vi "AM Modulation Demo (Baseband-Sine) - multi.vi"() -> ()   [LabVIEW 2013]
uses:
  <vilib>/express/express analysis/Spectral/Block/exnSpectralBlock spectral measurements power poly.vi
  <vilib>/express/express analysis/Spectral/Block/exnSpectralBlock spectral measurements power DDT.vi
  <vilib>/express/express analysis/Spectral/XNode/ExpressSpectralMeasurementsBlockNode.xnode
panel:
  in  "Noise Deviation":dbl=0.1 caption="Amplitude"
  out "After Filter 2":dynamicdata(graph)
  out "Baseband 2":dynamicdata(graph)
  out "Comparision 2":dynamicdata(graph)
  in  "DC Offset 2":dbl=1.0
  in  "Carrier Amp. 2":dbl=1.0 caption="Amplitude"
  in  "Carrier Freq. 2":dbl=100000.0 caption="Frequency"
  in  "Modulation Index 2":dbl(slide)=1.0 scale=0.0..5.0
  in  "Mod Freq. 2":dbl=1000.0 caption="Frequency"
  out "After Filter 1":dynamicdata(graph)
  in  "Mod Freq.":dbl=2000.0 caption="Frequency"
  in  "LPF Cut-Off":dbl=10000.0 caption="Lower Cut-Off"
  out "Comparision 1":dynamicdata(graph)
  out "Baseband 1":dynamicdata(graph)
  out "AM Power Spectrum":dynamicdata(graph)
  out "AM Wave":dynamicdata(graph)
  in  "DC Offset":dbl=1.0
  in  "Carrier Amp.":dbl=1.0 caption="Amplitude"
  in  "stop":bool
  in  "Modulation Index":dbl(slide)=1.0 scale=0.0..5.0
  in  "Carrier Freq.":dbl=50000.0 caption="Frequency"
  # "Amplitude Modulation"
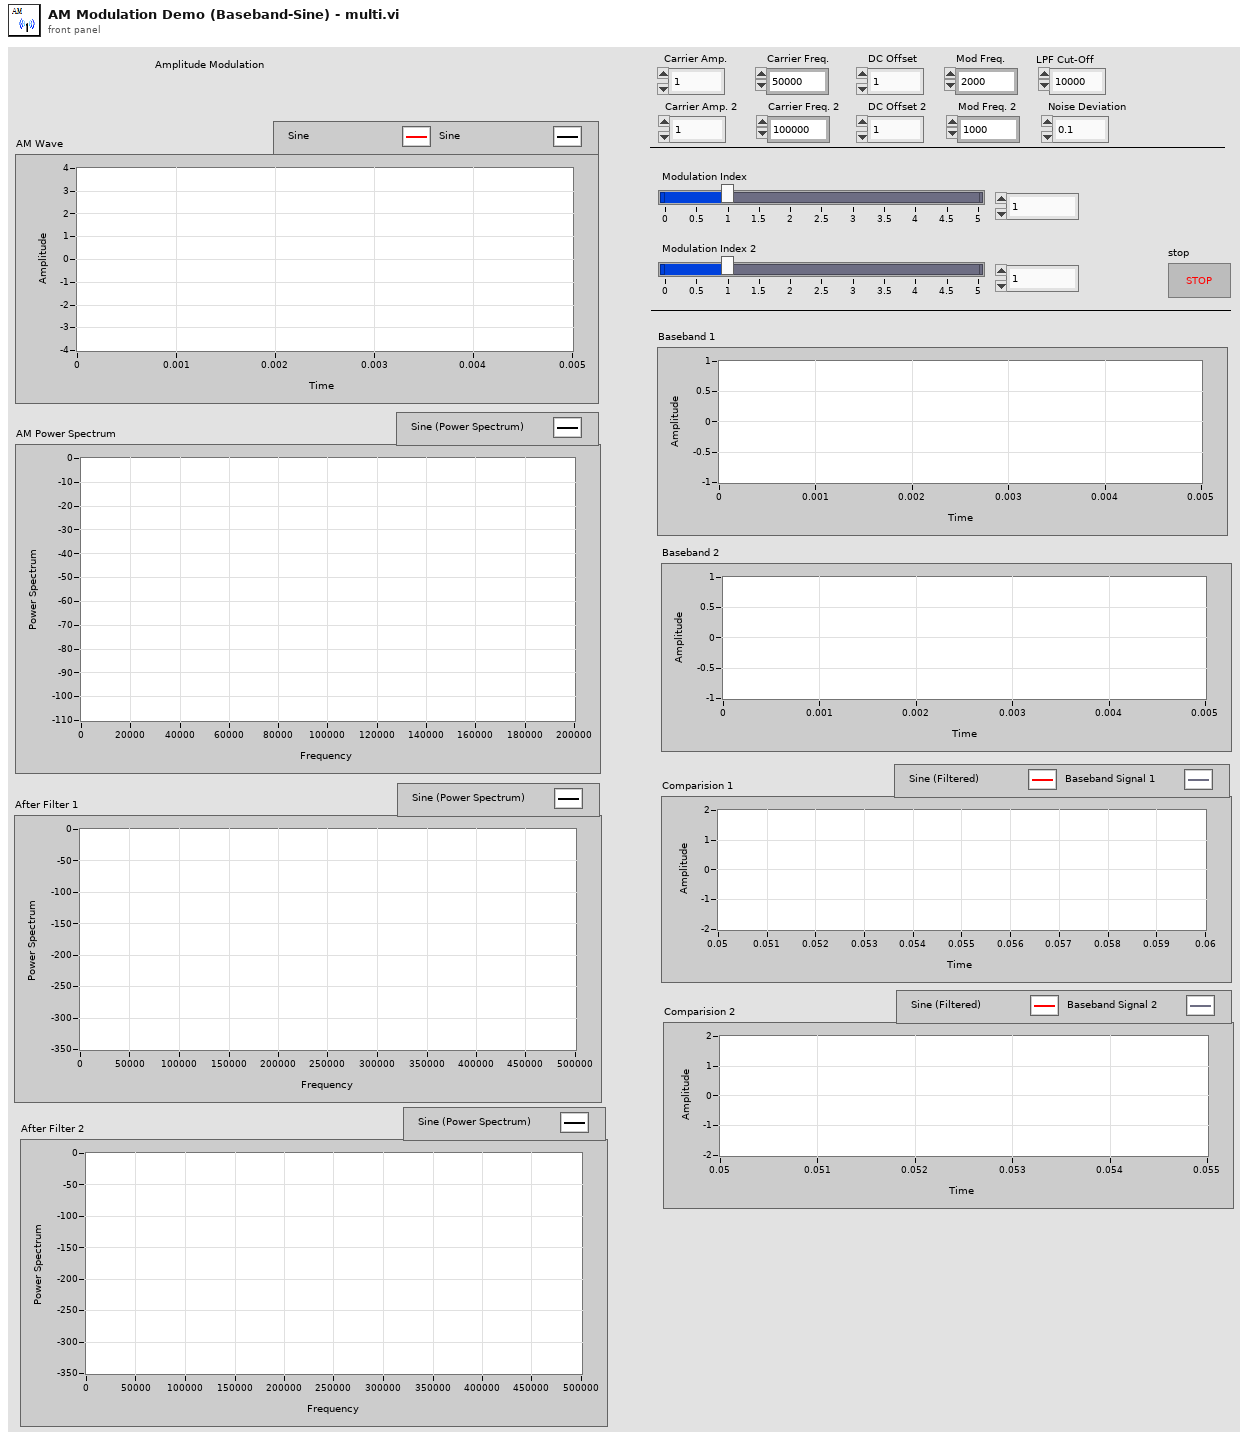
[diagram p1: front panel]
types:
  T1 = cluster{"averaging mode":u16, "weighting mode":u16, "number of averages":u32}
  T2 = cluster{"dB On (F)":bool, "unwrap phase (F)":bool, "convert to degree (F)":bool}
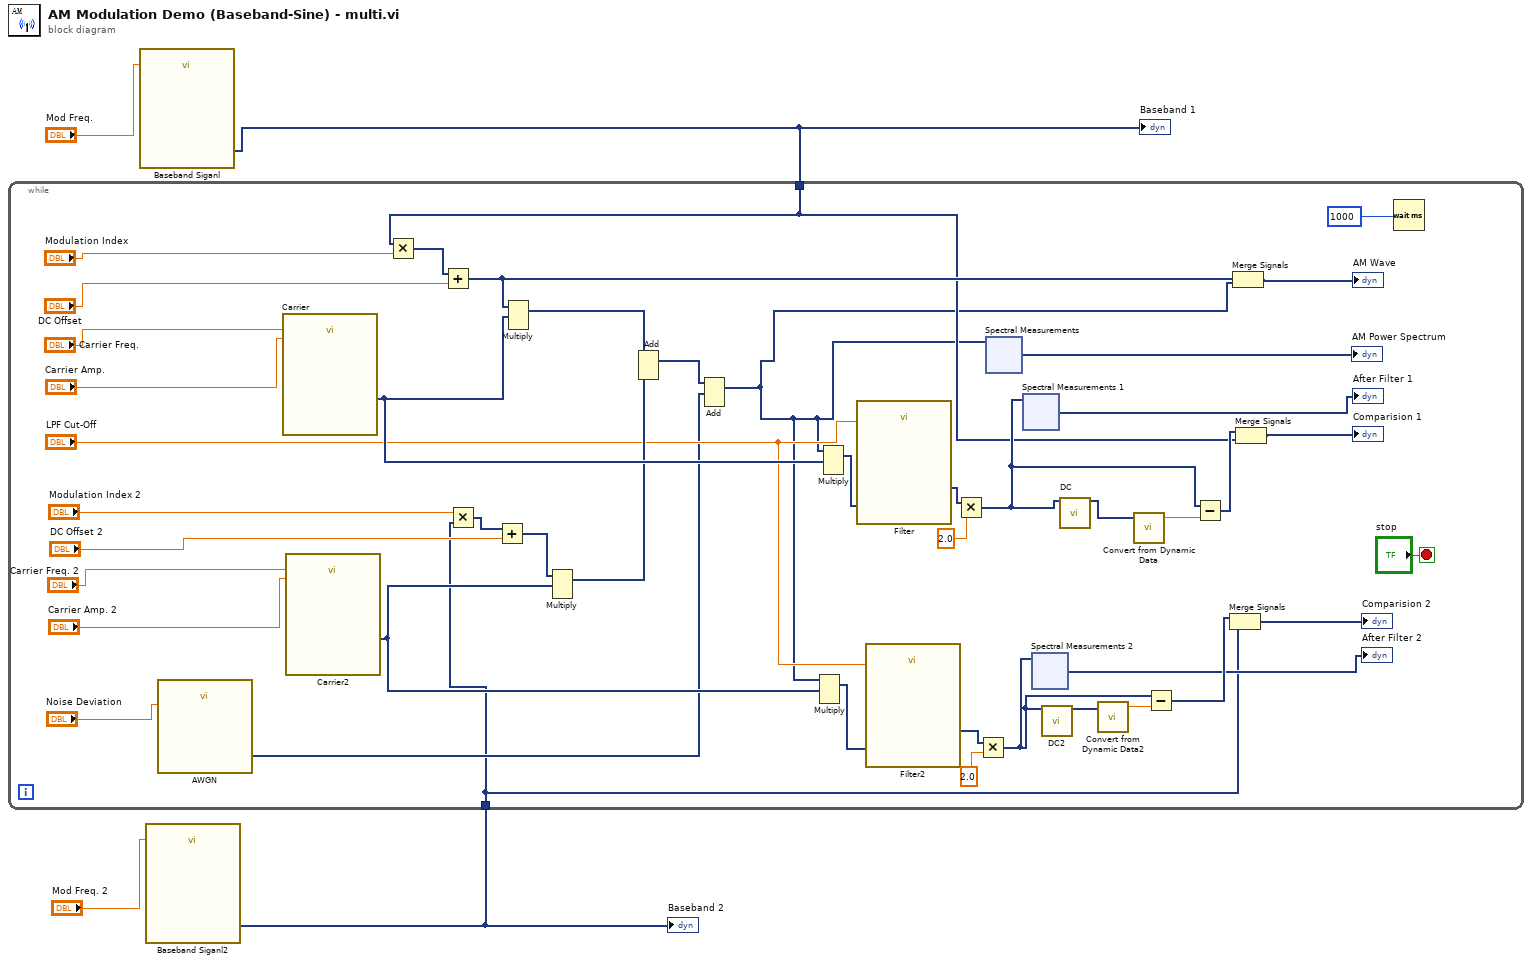
[diagram p0: block diagram]
diagram:
  n1 = call "Baseband Siganl"("Frequency"="Mod Freq.") -> ("Sine"=w3:dynamicdata)  [unwired: 13 in, 1 out]
  "Baseband 1" <- w3
  n2 = call "Baseband Siganl2"("Frequency"="Mod Freq. 2") -> ("Sine"=w1:dynamicdata)  [unwired: 13 in, 1 out]
  "Baseband 2" <- w1
  n3 = while {
    tunnel: w3 -> [w18]
    tunnel: w1 -> [w5]
    stop <- "stop" stop-if-true
    n4 = call "AWGN"("Standard deviation"="Noise Deviation") -> ("DC with Gaussian Noise"=w7:dynamicdata)  [unwired: 13 in, 1 out]
    n5 = call "Carrier"("Frequency"="Carrier Freq.", "Amplitude"="Carrier Amp.") -> ("Sine"=w25:dynamicdata)  [unwired: 12 in, 1 out]
    n6 = call "Carrier2"("Frequency"="Carrier Freq. 2", "Amplitude"="Carrier Amp. 2") -> ("Sine"=w16:dynamicdata)  [unwired: 12 in, 1 out]
    n7 = Multiply(x=w18, y="Modulation Index") -> (x*y=w47:dynamicdata)
    n8 = Add(x=w47, y="DC Offset") -> (x+y=w43:dynamicdata)
    n9 = Multiply(x="Modulation Index 2", y=w5) -> (x*y=w36:dynamicdata)
    n10 = Add(x=w36, y="DC Offset 2") -> (x+y=w34:dynamicdata)
    n11 = Multiply(1:w25, 2:w43) -> (0:w26:dynamicdata)  [unwired: 1 in, 1 out]
    n12 = Multiply(1:w16, 2:w34) -> (0:w17:dynamicdata)  [unwired: 1 in, 1 out]
    n13 = Add(1:w17, 2:w26) -> (0:w9:dynamicdata)  [unwired: 1 in, 1 out]
    n14 = Add(1:w7, 2:w9) -> (0:w8:dynamicdata)  [unwired: 1 in, 1 out]
    n15 = Multiply(1:w16, 2:w8) -> (0:w15:dynamicdata)  [unwired: 1 in, 1 out]
    n16 = Multiply(1:w25, 2:w8) -> (0:w29:dynamicdata)  [unwired: 1 in, 1 out]
    n17 = call "Filter"("Lower Cut-Off"="LPF Cut-Off", "Signal"=w29) -> ("Filtered Signal"=w28:dynamicdata)  [unwired: 8 in, 1 out]
    n18 = call "Filter2"("Lower Cut-Off"="LPF Cut-Off", "Signal"=w15) -> ("Filtered Signal"=w12:dynamicdata)  [unwired: 8 in, 1 out]
    n19 = Multiply(x=w28, y=2.0) -> (x*y=w20:dynamicdata)
    n20 = Multiply(x=w12, y=2.0) -> (x*y=w10:dynamicdata)
    n21 = xnode "Spectral Measurements"("Signals"=w8) -> ("Power Spectrum"=→"AM Power Spectrum":dynamicdata)  [unwired: 1 in, 1 out]
    n22 = xnode "Spectral Measurements 1"("Signals"=w20) -> ("Power Spectrum"=→"After Filter 1":dynamicdata)  [unwired: 1 in, 1 out]
    n23 = xnode "Spectral Measurements 2"("Signals"=w10) -> ("Power Spectrum"=→"After Filter 2":dynamicdata)  [unwired: 1 in, 1 out]
    n24 = call "DC2"("Signals"=w10) -> ("Mean (DC)"=w32:dynamicdata)  [unwired: 13 in, 1 out]
    n25 = call "DC"("Signals"=w20) -> ("Mean (DC)"=w22:dynamicdata)  [unwired: 13 in, 1 out]
    n26 = call "Convert from Dynamic Data2"("Dynamic Data Type"=w32) -> ("Scalar"=w31:dbl)  [unwired: 3 in]
    n27 = call "Convert from Dynamic Data"("Dynamic Data Type"=w22) -> ("Scalar"=w21:dbl)  [unwired: 3 in]
    n28 = Subtract(x=w10, y=w31) -> (x-y=w30:dynamicdata)
    n29 = Subtract(x=w20, y=w21) -> (x-y=w19:dynamicdata)
    n30 = Merge Signals(w30, w5) -> (→"Comparision 2":dynamicdata)
    n31 = Merge Signals(w43, w8) -> (→"AM Wave":dynamicdata)
    n32 = Merge Signals(w19, w18) -> (→"Comparision 1":dynamicdata)
    n33 = Wait (ms)(milliseconds to wait=1000) -> ()  [unwired: 1 out]
  }
